vi "test_RS-xxx to GPIB ConvBox Read.vi"(8 "error in (no error)":errorcluster, 11 "TestCase in":refnum<class "Instrument Addon Serial Protocols Unit Tests.lvclass">) -> (0 "error out":errorcluster, 3 "TestCase out":refnum<class "Instrument Addon Serial Protocols Unit Tests.lvclass">)   [LabVIEW 2023, in "Instrument Addon Serial Protocols Unit Tests.lvclass"]
uses:
  Instrument Addon Serial Protocols Unit Tests.lvclass
  Instrument Addon Serial Protocols Unit Tests.lvclass/Instrument Addon Serial Protocols Unit Tests.ctl
  <vilib>/addons/_JKI Toolkits/VI Tester/TestCase.llb/TestCase.lvclass
  Listener/ListenerClassControls/Operation.ctl
  Listener/Listener.lvclass
  RS-xxx to GPIB ConvBox/RS-xxx to GPIB ConvBox.lvclass
  <vilib>/platform/TimedLoop/XDataNode/XDataNode.xnode
  <vilib>/Platform/TimedLoop/XDataNode/nitl_modes.ctl
  <vilib>/Platform/TimedLoop/XDataNode/XDNodeRunTimeDep.lvlib
  <vilib>/Platform/TimedLoop/XDataNode/wakeup.ctl
  <vilib>/Platform/TimedLoop/XDataNode/timing_clust.ctl
  Protocol Parent/Methods/Read Parameter.ctl
  Protocol Parent/Protocol Parent.lvclass
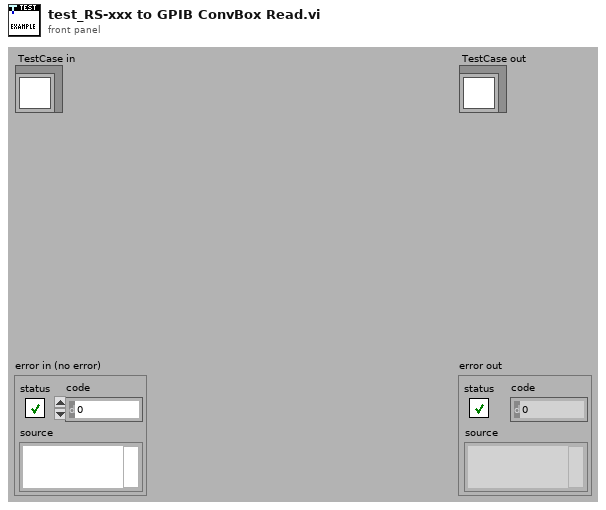
[diagram p1: front panel]
types:
  T1 = typedef "Protocols.lvlib/Protocol Parent.lvclass/Read Parameter.ctl" = cluster{"Wait Type":enum16{"Byte Count", "Wait sec"}, "Wait Value":dbl}
  T2 = typedef "Listener.lvclass/Operation.ctl" = enum16{"Read", "Write"}
  T3 = typedef "XDNodeRunTimeDep.lvlib/timing_clust.ctl" = cluster{"Expected End [f-1]":u64, "Actual End [f-1]":u64, "Finished Late? [f-1]":bool, "Expected End [i-1]":u64, "Actual End [i-1]":u64, "Finished Late? [i-1]":bool, "Expected Start [i]":u64, "Actual Start [i]":u64, "Expected Start [f]":u64, "Actual Start [f]":u64, "Source Name":string, "Structure Name":string, "Period":i64, "Deadline":i64, "Offset":i64, "Start":i64, "Priority":i32, "Timeout":i32, "Mode":T4, "Wakeup Reason":T5, "Error":errorcluster, "Source Type":string, "Secondary Source Type":string, "Global End Time":u64, "Global Start Time":u64, "Frame Duration":u64, "Iteration Duration":u64, "Assigned CPU":i32, "I/O Scan Engine Mode":u32}
  T4 = typedef "XDNodeRunTimeDep.lvlib/nitl_modes.ctl" = enum32{"No Change", "Process missed periods, maintain original phase", "Discard missed periods, maintain original phase", "Process missed periods, ignore original phase", "Discard missed periods, ignore original phase"}
  T5 = typedef "XDNodeRunTimeDep.lvlib/wakeup.ctl" = enum32{"Normal", "Aborted", "Asynchronous wakeup", "Timing source error", "Timed loop error", "Timeout"}
  T6 = typedef "Listener.lvclass/RS-xxx To GPIB ConvBox Data Structure.ctl" = cluster{"Data":string, "Command Messages Read":string[], "Address":string, "Data Length":u32}
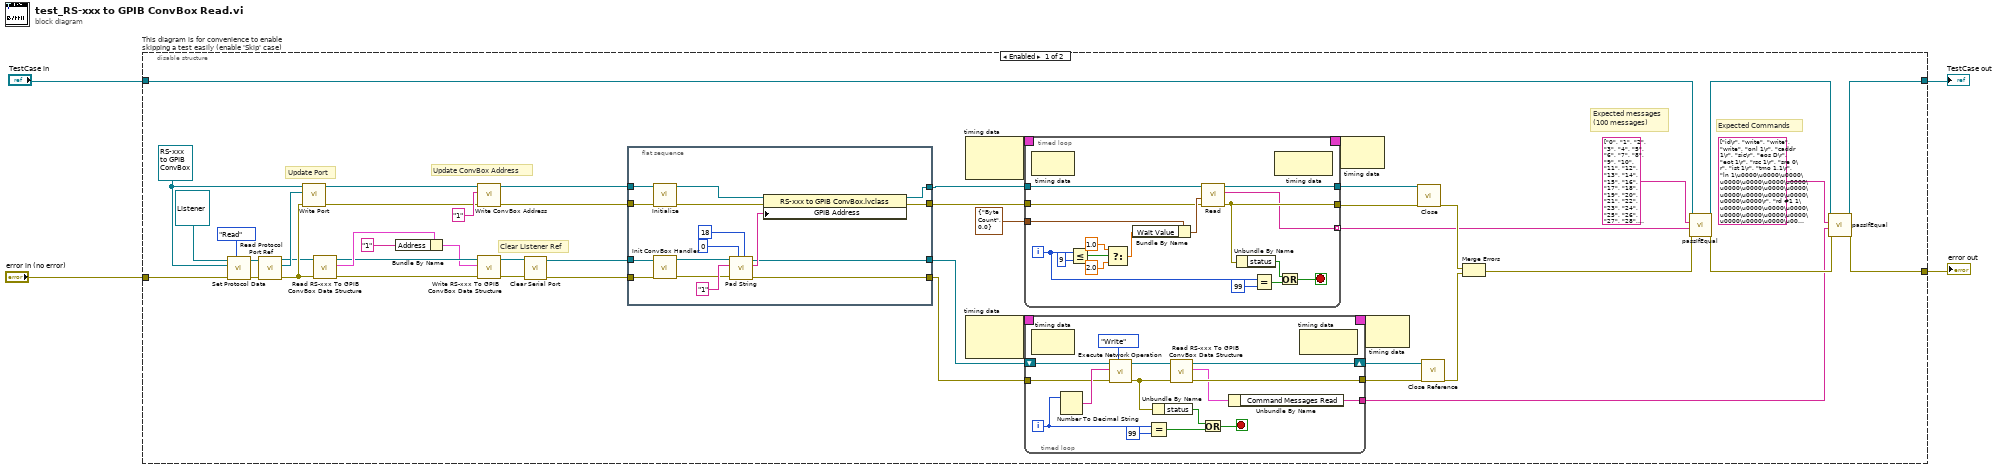
[diagram p0: block diagram]
diagram:
  n1 = disable-structure "This diagram is for convenience to enable skipping a test easily (enable 'Skip' case)" shown="Enabled" {
    disable-tunnel: "TestCase in" -> [w52 w112]
    disable-tunnel: [w10 w110] -> w1
    disable-tunnel: [w12 w111] -> w3
    disable-tunnel: "error in (no error)" -> [w51 w109]
    frame Enabled {
      w43 = refnum<class "RS-xxx to GPIB ConvBox.lvclass"> refnum ("Protocols.lvlib:RS-xxx to GPIB ConvBox.lvclass")
      # "Expected Commands"
      # "Update Port"
      # "Expected messages\n(100 messages)"
      # "Update ConvBox Address"
      # "Clear Listener Ref"
      n2 = call "Set Protocol Data.vi"("Operation"=Operation."Read", "error in (no error)"=w51, "Protocols.lvlib:Protocol Parent.lvclass"=w43, "Listener In.lvclass"=refnum<class "Listener.lvclass"> refnum ("Listener.lvclass")) -> ("error out"=w47:errorcluster, "Listener Out.lvclass"=w46:refnum<class "Listener.lvclass">)  [unwired: 6 in]
      n3 = call "Read Protocol Port Ref.vi"("error in (no error)"=w47, "Listener in"=w46) -> ("error out"=w29:errorcluster, "Protocol Port Ref"=w42:refnum<visa-resource-name>, "Listener out"=w28:refnum<class "Listener.lvclass">)  [unwired: 7 in]
      n4 = call "Write Port.vi"("error in (no error)"=w29, "Port"=w42, "RS232 to GPIB ConvBox in"=w43) -> ("error out"=w45:errorcluster, "RS232 to GPIB ConvBox out"=w44:refnum<class "RS-xxx to GPIB ConvBox.lvclass">)  [unwired: 7 in]
      n5 = call-dynamic "Read RS-xxx To GPIB ConvBox Data Structure.vi"("error in (no error)"=w29, "Listener in"=w28) -> ("error out"=w24:errorcluster, "RS-xxx To GPIB ConvBox Data Structure"=w27:T6, "Listener out"=w25:refnum<class "Listener.lvclass">)  [unwired: 7 in]
      n6 = Bundle By Name(cluster=w27, "Address"="1") -> (w23:T6)
      n7 = call "Write ConvBox Address.vi"("error in (no error)"=w45, "ConvBox Address"="1", "RS232 to GPIB ConvBox in"=w44) -> ("error out"=w8:errorcluster, "RS232 to GPIB ConvBox out"=w7:refnum<class "RS-xxx to GPIB ConvBox.lvclass">)  [unwired: 7 in]
      n8 = call-dynamic "Write RS-xxx To GPIB ConvBox Data Structure.vi"("error in (no error)"=w24, "RS-xxx To GPIB ConvBox Data Structure"=w23, "Listener in"=w25) -> ("error out"=w22:errorcluster, "Listener out"=w21:refnum<class "Listener.lvclass">)  [unwired: 7 in]
      n9 = call "Clear Serial Port.vi"("error in (no error)"=w22, "Listener In.lvclass"=w21) -> ("error out"=w6:errorcluster, "Listener out"=w5:refnum<class "Listener.lvclass">)  [unwired: 8 in]
      n10 = flat-sequence {
        tunnel: [w64] -> w20
        tunnel: [w63] -> w19
        tunnel: [w62] -> w18
        tunnel: [w61] -> w17
        tunnel: w8 -> [w60]
        tunnel: w7 -> [w59]
        tunnel: w6 -> [w56]
        tunnel: w5 -> [w55]
        frame #0 {
          n11 = call-dynamic "Initialize.vi"("error in (no error)"=w60, "RS232 to GPIB ConvBox in"=w59) -> ("error out"=w58:errorcluster, "RS232 to GPIB ConvBox out"=w57:refnum<class "RS-xxx to GPIB ConvBox.lvclass">)  [unwired: 8 in]
          n12 = call "Init ConvBox Handler.vi"("error in (no error)"=w56, "Listener in"=w55) -> ("error out"=w54:errorcluster, "Listener out"=w53:refnum<class "Listener.lvclass">)  [unwired: 8 in]
          n13 = call "Pad String.vi"("Expected Length"=u8 18, "Pad Character"=u8 0, "error in (no error)"=w54, "String To Pad"="1", "Listener in"=w53) -> ("error out"=w62:errorcluster, "Padded String"=w65:string, "Listener out"=w61:refnum<class "Listener.lvclass">)  [unwired: 4 in]
          n14 = property class="RS-xxx to GPIB ConvBox.lvclass"(reference=w57, error in=w58, "GPIB Address"=w65) -> (reference out=w63:refnum<class "RS-xxx to GPIB ConvBox.lvclass">, error out=w64:errorcluster)
        }
      }
      n15 = node-c288() -> (w41:T3)  [unwired: 2 in]
      n16 = node-c288() -> (w38:T3)  [unwired: 2 in]
      n17 = timed-loop {
        timing: w41 -> [_]
        timing-out: [_] -> w40
        tunnel: T1 {"Wait Type"=enum."Byte Count", "Wait Value"=0.0} ("Read Parameter") -> [w99]
        tunnel: [w96] -> w34
        tunnel: [w95] -> w33
        tunnel: [w94] -> w15 mode=indexing
        tunnel: w20 -> [w92]
        tunnel: w19 -> [w93]
        i -> [w90]
        stop <- w87 stop-if-true
        n18 = node-c288() -> ()  [unwired: 1 in, 1 out]
        n19 = Less Or Equal?(x=w90, y=9) -> (x <= y?=w102:bool)
        n20 = Select(t=1.0, s=w102, f=2.0) -> (s? t:f=w98:dbl)
        n21 = Bundle By Name(cluster=w99, "Wait Value"=w98) -> (w97:T1)
        n22 = call-dynamic "Read.vi"("error in (no error)"=w92, "Variant"=w97, "RS232 to GPIB ConvBox in"=w93) -> ("error out"=w96:errorcluster, "String"=w94:string, "RS232 to GPIB ConvBox out"=w95:refnum<class "RS-xxx to GPIB ConvBox.lvclass">)  [unwired: 6 in]
        n23 = Unbundle By Name(w96) -> ("status"=w91:bool)
        n24 = Equal?(x=w90, y=99) -> (x = y?=w88:bool)
        n25 = node-c288() -> ()  [unwired: 1 in, 1 out]
        n26 = Or(x=w91, y=w88) -> (x .or. y?=w87:bool)
      }
      n27 = timed-loop {
        timing: w38 -> [_]
        timing-out: [_] -> w37
        tunnel: [w71] -> w36
        tunnel: w18 -> [w81]
        tunnel: [w69] -> w13
        shift-right: [w72] -> w35
        shift-left: w17 -> [w80]
        i -> [w77]
        stop <- w78 stop-if-true
        n28 = node-c288() -> ()  [unwired: 1 in, 1 out]
        n29 = Number To Decimal String(number=w77) -> (decimal integer string=w82:string)  [unwired: 1 in]
        n30 = call "Execute Network Operation.vi"("Operation"=Operation."Write", "error in (no error)"=w81, "Message"=w82, "Listener In.lvclass"=w80) -> ("error out"=w73:errorcluster, "Listener Out.lvclass"=w74:refnum<class "Listener.lvclass">)  [unwired: 6 in]
        n31 = Equal?(x=w77, y=99) -> (x = y?=w75:bool)
        n32 = Unbundle By Name(w73) -> ("status"=w79:bool)
        n33 = call-dynamic "Read RS-xxx To GPIB ConvBox Data Structure.vi"("error in (no error)"=w73, "Listener in"=w74) -> ("error out"=w71:errorcluster, "RS-xxx To GPIB ConvBox Data Structure"=w70:T6, "Listener out"=w72:refnum<class "Listener.lvclass">)  [unwired: 7 in]
        n34 = Or(x=w79, y=w75) -> (x .or. y?=w78:bool)
        n35 = Unbundle By Name(w70) -> ("Command Messages Read"=w69:string[])
        n36 = node-c288() -> ()  [unwired: 1 in, 1 out]
      }
      n37 = node-c288(w40) -> ()  [unwired: 1 out]
      n38 = node-c288(w37) -> ()  [unwired: 1 out]
      n39 = call-dynamic "Close.vi"("error in (no error)"=w34, "RS232 to GPIB ConvBox in"=w33) -> ("error out"=w32:errorcluster)  [unwired: 8 in, 1 out]
      n40 = call "Close Reference.vi"("error in (no error)"=w36, "Listener In.lvclass"=w35) -> ("error out"=w31:errorcluster)  [unwired: 8 in, 1 out]
      n41 = Merge Errors(w32, w31) -> (w30:errorcluster)
      n42 = call-dynamic "passIfEqual.vi"("error in (no error)"=w30, "y"=w15, "x"=string[] ["0", "1", "2", "3", "4", "5", "6", "7", "8", "9", "10", "11", "12", "13", "14", "15", "16", "17", "18", "19", "20", "21", "22", "23", "24", "25", "26", "27", "28", "29", "30", "31", "32", "33", "34", "35", "36", "37", "38", "39", "40", "41", "42", "43", "44", "45", "46", "47", "48", "49", "50", "51", "52", "53", "54", "55", "56", "57", "58", "59", "60", "61", "62", "63", "64", "65", "66", "67", "68", "69", "70", "71", "72", "73", "74", "75", "76", "77", "78", "79", "80", "81", "82", "83", "84", "85", "86", "87", "88", "89", "90", "91", "92", "93", "94", "95", "96", "97", "98", "99"] ("Array"), "TestCase in"=w52) -> ("error out"=w14:errorcluster, "TestCase out"=w11:refnum<class "Instrument Addon Serial Protocols Unit Tests.lvclass">)  [unwired: 6 in]
      n43 = call-dynamic "passIfEqual.vi"("error in (no error)"=w14, "y"=w13, "x"=string[] ["id\r", "write", "write", "write", "onl 1\r", "caddr 1\r", "sic\r", "eos D\r", "eot 1\r", "rsc 1\r", "sre 0\r", "ist 1\r", "tmo 1,1\r", "ln 1\u0000\u0000\u0000\u0000\u0000\u0000\u0000\u0000\u0000\u0000\u0000\u0000\u0000\u0000\u0000\u0000\u0000\r", "rd #1 1\u0000\u0000\u0000\u0000\u0000\u0000\u0000\u0000\u0000\u0000\u0000\u0000\u0000\u0000\u0000\u0000\u0000\r", "stat n\r", "ln 1\u0000\u0000\u0000\u0000\u0000\u0000\u0000\u0000\u0000\u0000\u0000\u0000\u0000\u0000\u0000\u0000\u0000\r", "rd #1 1\u0000\u0000\u0000\u0000\u0000\u0000\u0000\u0000\u0000\u0000\u0000\u0000\u0000\u0000\u0000\u0000\u0000\r", "stat n\r", "ln 1\u0000\u0000\u0000\u0000\u0000\u0000\u0000\u0000\u0000\u0000\u0000\u0000\u0000\u0000\u0000\u0000\u0000\r", "rd #1 1\u0000\u0000\u0000\u0000\u0000\u0000\u0000\u0000\u0000\u0000\u0000\u0000\u0000\u0000\u0000\u0000\u0000\r", "stat n\r", "ln 1\u0000\u0000\u0000\u0000\u0000\u0000\u0000\u0000\u0000\u0000\u0000\u0000\u0000\u0000\u0000\u0000\u0000\r", "rd #1 1\u0000\u0000\u0000\u0000\u0000\u0000\u0000\u0000\u0000\u0000\u0000\u0000\u0000\u0000\u0000\u0000\u0000\r", "stat n\r", "ln 1\u0000\u0000\u0000\u0000\u0000\u0000\u0000\u0000\u0000\u0000\u0000\u0000\u0000\u0000\u0000\u0000\u0000\r", "rd #1 1\u0000\u0000\u0000\u0000\u0000\u0000\u0000\u0000\u0000\u0000\u0000\u0000\u0000\u0000\u0000\u0000\u0000\r", "stat n\r", "ln 1\u0000\u0000\u0000\u0000\u0000\u0000\u0000\u0000\u0000\u0000\u0000\u0000\u0000\u0000\u0000\u0000\u0000\r", "rd #1 1\u0000\u0000\u0000\u0000\u0000\u0000\u0000\u0000\u0000\u0000\u0000\u0000\u0000\u0000\u0000\u0000\u0000\r", "stat n\r", "ln 1\u0000\u0000\u0000\u0000\u0000\u0000\u0000\u0000\u0000\u0000\u0000\u0000\u0000\u0000\u0000\u0000\u0000\r", "rd #1 1\u0000\u0000\u0000\u0000\u0000\u0000\u0000\u0000\u0000\u0000\u0000\u0000\u0000\u0000\u0000\u0000\u0000\r", "stat n\r", "ln 1\u0000\u0000\u0000\u0000\u0000\u0000\u0000\u0000\u0000\u0000\u0000\u0000\u0000\u0000\u0000\u0000\u0000\r", "rd #1 1\u0000\u0000\u0000\u0000\u0000\u0000\u0000\u0000\u0000\u0000\u0000\u0000\u0000\u0000\u0000\u0000\u0000\r", "stat n\r", "ln 1\u0000\u0000\u0000\u0000\u0000\u0000\u0000\u0000\u0000\u0000\u0000\u0000\u0000\u0000\u0000\u0000\u0000\r", "rd #1 1\u0000\u0000\u0000\u0000\u0000\u0000\u0000\u0000\u0000\u0000\u0000\u0000\u0000\u0000\u0000\u0000\u0000\r", "stat n\r", "ln 1\u0000\u0000\u0000\u0000\u0000\u0000\u0000\u0000\u0000\u0000\u0000\u0000\u0000\u0000\u0000\u0000\u0000\r", "rd #1 1\u0000\u0000\u0000\u0000\u0000\u0000\u0000\u0000\u0000\u0000\u0000\u0000\u0000\u0000\u0000\u0000\u0000\r", "stat n\r", "ln 1\u0000\u0000\u0000\u0000\u0000\u0000\u0000\u0000\u0000\u0000\u0000\u0000\u0000\u0000\u0000\u0000\u0000\r", "rd #2 1\u0000\u0000\u0000\u0000\u0000\u0000\u0000\u0000\u0000\u0000\u0000\u0000\u0000\u0000\u0000\u0000\u0000\r", "stat n\r", "ln 1\u0000\u0000\u0000\u0000\u0000\u0000\u0000\u0000\u0000\u0000\u0000\u0000\u0000\u0000\u0000\u0000\u0000\r", "rd #2 1\u0000\u0000\u0000\u0000\u0000\u0000\u0000\u0000\u0000\u0000\u0000\u0000\u0000\u0000\u0000\u0000\u0000\r", "stat n\r", "ln 1\u0000\u0000\u0000\u0000\u0000\u0000\u0000\u0000\u0000\u0000\u0000\u0000\u0000\u0000\u0000\u0000\u0000\r", "rd #2 1\u0000\u0000\u0000\u0000\u0000\u0000\u0000\u0000\u0000\u0000\u0000\u0000\u0000\u0000\u0000\u0000\u0000\r", "stat n\r", "ln 1\u0000\u0000\u0000\u0000\u0000\u0000\u0000\u0000\u0000\u0000\u0000\u0000\u0000\u0000\u0000\u0000\u0000\r", "rd #2 1\u0000\u0000\u0000\u0000\u0000\u0000\u0000\u0000\u0000\u0000\u0000\u0000\u0000\u0000\u0000\u0000\u0000\r", "stat n\r", "ln 1\u0000\u0000\u0000\u0000\u0000\u0000\u0000\u0000\u0000\u0000\u0000\u0000\u0000\u0000\u0000\u0000\u0000\r", "rd #2 1\u0000\u0000\u0000\u0000\u0000\u0000\u0000\u0000\u0000\u0000\u0000\u0000\u0000\u0000\u0000\u0000\u0000\r", "stat n\r", "ln 1\u0000\u0000\u0000\u0000\u0000\u0000\u0000\u0000\u0000\u0000\u0000\u0000\u0000\u0000\u0000\u0000\u0000\r", "rd #2 1\u0000\u0000\u0000\u0000\u0000\u0000\u0000\u0000\u0000\u0000\u0000\u0000\u0000\u0000\u0000\u0000\u0000\r", "stat n\r", "ln 1\u0000\u0000\u0000\u0000\u0000\u0000\u0000\u0000\u0000\u0000\u0000\u0000\u0000\u0000\u0000\u0000\u0000\r", "rd #2 1\u0000\u0000\u0000\u0000\u0000\u0000\u0000\u0000\u0000\u0000\u0000\u0000\u0000\u0000\u0000\u0000\u0000\r", "stat n\r", "ln 1\u0000\u0000\u0000\u0000\u0000\u0000\u0000\u0000\u0000\u0000\u0000\u0000\u0000\u0000\u0000\u0000\u0000\r", "rd #2 1\u0000\u0000\u0000\u0000\u0000\u0000\u0000\u0000\u0000\u0000\u0000\u0000\u0000\u0000\u0000\u0000\u0000\r", "stat n\r", "ln 1\u0000\u0000\u0000\u0000\u0000\u0000\u0000\u0000\u0000\u0000\u0000\u0000\u0000\u0000\u0000\u0000\u0000\r", "rd #2 1\u0000\u0000\u0000\u0000\u0000\u0000\u0000\u0000\u0000\u0000\u0000\u0000\u0000\u0000\u0000\u0000\u0000\r", "stat n\r", "ln 1\u0000\u0000\u0000\u0000\u0000\u0000\u0000\u0000\u0000\u0000\u0000\u0000\u0000\u0000\u0000\u0000\u0000\r", "rd #2 1\u0000\u0000\u0000\u0000\u0000\u0000\u0000\u0000\u0000\u0000\u0000\u0000\u0000\u0000\u0000\u0000\u0000\r", "stat n\r", "ln 1\u0000\u0000\u0000\u0000\u0000\u0000\u0000\u0000\u0000\u0000\u0000\u0000\u0000\u0000\u0000\u0000\u0000\r", "rd #2 1\u0000\u0000\u0000\u0000\u0000\u0000\u0000\u0000\u0000\u0000\u0000\u0000\u0000\u0000\u0000\u0000\u0000\r", "stat n\r", "ln 1\u0000\u0000\u0000\u0000\u0000\u0000\u0000\u0000\u0000\u0000\u0000\u0000\u0000\u0000\u0000\u0000\u0000\r", "rd #2 1\u0000\u0000\u0000\u0000\u0000\u0000\u0000\u0000\u0000\u0000\u0000\u0000\u0000\u0000\u0000\u0000\u0000\r", "stat n\r", "ln 1\u0000\u0000\u0000\u0000\u0000\u0000\u0000\u0000\u0000\u0000\u0000\u0000\u0000\u0000\u0000\u0000\u0000\r", "rd #2 1\u0000\u0000\u0000\u0000\u0000\u0000\u0000\u0000\u0000\u0000\u0000\u0000\u0000\u0000\u0000\u0000\u0000\r", "stat n\r", "ln 1\u0000\u0000\u0000\u0000\u0000\u0000\u0000\u0000\u0000\u0000\u0000\u0000\u0000\u0000\u0000\u0000\u0000\r", "rd #2 1\u0000\u0000\u0000\u0000\u0000\u0000\u0000\u0000\u0000\u0000\u0000\u0000\u0000\u0000\u0000\u0000\u0000\r", "stat n\r", "ln 1\u0000\u0000\u0000\u0000\u0000\u0000\u0000\u0000\u0000\u0000\u0000\u0000\u0000\u0000\u0000\u0000\u0000\r", "rd #2 1\u0000\u0000\u0000\u0000\u0000\u0000\u0000\u0000\u0000\u0000\u0000\u0000\u0000\u0000\u0000\u0000\u0000\r", "stat n\r", "ln 1\u0000\u0000\u0000\u0000\u0000\u0000\u0000\u0000\u0000\u0000\u0000\u0000\u0000\u0000\u0000\u0000\u0000\r", "rd #2 1\u0000\u0000\u0000\u0000\u0000\u0000\u0000\u0000\u0000\u0000\u0000\u0000\u0000\u0000\u0000\u0000\u0000\r", "stat n\r", "ln 1\u0000\u0000\u0000\u0000\u0000\u0000\u0000\u0000\u0000\u0000\u0000\u0000\u0000\u0000\u0000\u0000\u0000\r", "rd #2 1\u0000\u0000\u0000\u0000\u0000\u0000\u0000\u0000\u0000\u0000\u0000\u0000\u0000\u0000\u0000\u0000\u0000\r", "stat n\r", "ln 1\u0000\u0000\u0000\u0000\u0000\u0000\u0000\u0000\u0000\u0000\u0000\u0000\u0000\u0000\u0000\u0000\u0000\r", "rd #2 1\u0000\u0000\u0000\u0000\u0000\u0000\u0000\u0000\u0000\u0000\u0000\u0000\u0000\u0000\u0000\u0000\u0000\r", "stat n\r", "ln 1\u0000\u0000\u0000\u0000\u0000\u0000\u0000\u0000\u0000\u0000\u0000\u0000\u0000\u0000\u0000\u0000\u0000\r", "rd #2 1\u0000\u0000\u0000\u0000\u0000\u0000\u0000\u0000\u0000\u0000\u0000\u0000\u0000\u0000\u0000\u0000\u0000\r", "stat n\r", "ln 1\u0000\u0000\u0000\u0000\u0000\u0000\u0000\u0000\u0000\u0000\u0000\u0000\u0000\u0000\u0000\u0000\u0000\r", "rd #2 1\u0000\u0000\u0000\u0000\u0000\u0000\u0000\u0000\u0000\u0000\u0000\u0000\u0000\u0000\u0000\u0000\u0000\r", "stat n\r", "ln 1\u0000\u0000\u0000\u0000\u0000\u0000\u0000\u0000\u0000\u0000\u0000\u0000\u0000\u0000\u0000\u0000\u0000\r", "rd #2 1\u0000\u0000\u0000\u0000\u0000\u0000\u0000\u0000\u0000\u0000\u0000\u0000\u0000\u0000\u0000\u0000\u0000\r", "stat n\r", "ln 1\u0000\u0000\u0000\u0000\u0000\u0000\u0000\u0000\u0000\u0000\u0000\u0000\u0000\u0000\u0000\u0000\u0000\r", "rd #2 1\u0000\u0000\u0000\u0000\u0000\u0000\u0000\u0000\u0000\u0000\u0000\u0000\u0000\u0000\u0000\u0000\u0000\r", "stat n\r", "ln 1\u0000\u0000\u0000\u0000\u0000\u0000\u0000\u0000\u0000\u0000\u0000\u0000\u0000\u0000\u0000\u0000\u0000\r", "rd #2 1\u0000\u0000\u0000\u0000\u0000\u0000\u0000\u0000\u0000\u0000\u0000\u0000\u0000\u0000\u0000\u0000\u0000\r", "stat n\r", "ln 1\u0000\u0000\u0000\u0000\u0000\u0000\u0000\u0000\u0000\u0000\u0000\u0000\u0000\u0000\u0000\u0000\u0000\r", "rd #2 1\u0000\u0000\u0000\u0000\u0000\u0000\u0000\u0000\u0000\u0000\u0000\u0000\u0000\u0000\u0000\u0000\u0000\r", "stat n\r", "ln 1\u0000\u0000\u0000\u0000\u0000\u0000\u0000\u0000\u0000\u0000\u0000\u0000\u0000\u0000\u0000\u0000\u0000\r", "rd #2 1\u0000\u0000\u0000\u0000\u0000\u0000\u0000\u0000\u0000\u0000\u0000\u0000\u0000\u0000\u0000\u0000\u0000\r", "stat n\r", "ln 1\u0000\u0000\u0000\u0000\u0000\u0000\u0000\u0000\u0000\u0000\u0000\u0000\u0000\u0000\u0000\u0000\u0000\r", "rd #2 1\u0000\u0000\u0000\u0000\u0000\u0000\u0000\u0000\u0000\u0000\u0000\u0000\u0000\u0000\u0000\u0000\u0000\r", "stat n\r", "ln 1\u0000\u0000\u0000\u0000\u0000\u0000\u0000\u0000\u0000\u0000\u0000\u0000\u0000\u0000\u0000\u0000\u0000\r", "rd #2 1\u0000\u0000\u0000\u0000\u0000\u0000\u0000\u0000\u0000\u0000\u0000\u0000\u0000\u0000\u0000\u0000\u0000\r", "stat n\r", "ln 1\u0000\u0000\u0000\u0000\u0000\u0000\u0000\u0000\u0000\u0000\u0000\u0000\u0000\u0000\u0000\u0000\u0000\r", "rd #2 1\u0000\u0000\u0000\u0000\u0000\u0000\u0000\u0000\u0000\u0000\u0000\u0000\u0000\u0000\u0000\u0000\u0000\r", "stat n\r", "ln 1\u0000\u0000\u0000\u0000\u0000\u0000\u0000\u0000\u0000\u0000\u0000\u0000\u0000\u0000\u0000\u0000\u0000\r", "rd #2 1\u0000\u0000\u0000\u0000\u0000\u0000\u0000\u0000\u0000\u0000\u0000\u0000\u0000\u0000\u0000\u0000\u0000\r", "stat n\r", "ln 1\u0000\u0000\u0000\u0000\u0000\u0000\u0000\u0000\u0000\u0000\u0000\u0000\u0000\u0000\u0000\u0000\u0000\r", "rd #2 1\u0000\u0000\u0000\u0000\u0000\u0000\u0000\u0000\u0000\u0000\u0000\u0000\u0000\u0000\u0000\u0000\u0000\r", "stat n\r", "ln 1\u0000\u0000\u0000\u0000\u0000\u0000\u0000\u0000\u0000\u0000\u0000\u0000\u0000\u0000\u0000\u0000\u0000\r", "rd #2 1\u0000\u0000\u0000\u0000\u0000\u0000\u0000\u0000\u0000\u0000\u0000\u0000\u0000\u0000\u0000\u0000\u0000\r", "stat n\r", "ln 1\u0000\u0000\u0000\u0000\u0000\u0000\u0000\u0000\u0000\u0000\u0000\u0000\u0000\u0000\u0000\u0000\u0000\r", "rd #2 1\u0000\u0000\u0000\u0000\u0000\u0000\u0000\u0000\u0000\u0000\u0000\u0000\u0000\u0000\u0000\u0000\u0000\r", "stat n\r", "ln 1\u0000\u0000\u0000\u0000\u0000\u0000\u0000\u0000\u0000\u0000\u0000\u0000\u0000\u0000\u0000\u0000\u0000\r", "rd #2 1\u0000\u0000\u0000\u0000\u0000\u0000\u0000\u0000\u0000\u0000\u0000\u0000\u0000\u0000\u0000\u0000\u0000\r", "stat n\r", "ln 1\u0000\u0000\u0000\u0000\u0000\u0000\u0000\u0000\u0000\u0000\u0000\u0000\u0000\u0000\u0000\u0000\u0000\r", "rd #2 1\u0000\u0000\u0000\u0000\u0000\u0000\u0000\u0000\u0000\u0000\u0000\u0000\u0000\u0000\u0000\u0000\u0000\r", "stat n\r", "ln 1\u0000\u0000\u0000\u0000\u0000\u0000\u0000\u0000\u0000\u0000\u0000\u0000\u0000\u0000\u0000\u0000\u0000\r", "rd #2 1\u0000\u0000\u0000\u0000\u0000\u0000\u0000\u0000\u0000\u0000\u0000\u0000\u0000\u0000\u0000\u0000\u0000\r", "stat n\r", "ln 1\u0000\u0000\u0000\u0000\u0000\u0000\u0000\u0000\u0000\u0000\u0000\u0000\u0000\u0000\u0000\u0000\u0000\r", "rd #2 1\u0000\u0000\u0000\u0000\u0000\u0000\u0000\u0000\u0000\u0000\u0000\u0000\u0000\u0000\u0000\u0000\u0000\r", "stat n\r", "ln 1\u0000\u0000\u0000\u0000\u0000\u0000\u0000\u0000\u0000\u0000\u0000\u0000\u0000\u0000\u0000\u0000\u0000\r", "rd #2 1\u0000\u0000\u0000\u0000\u0000\u0000\u0000\u0000\u0000\u0000\u0000\u0000\u0000\u0000\u0000\u0000\u0000\r", "stat n\r", "ln 1\u0000\u0000\u0000\u0000\u0000\u0000\u0000\u0000\u0000\u0000\u0000\u0000\u0000\u0000\u0000\u0000\u0000\r", "rd #2 1\u0000\u0000\u0000\u0000\u0000\u0000\u0000\u0000\u0000\u0000\u0000\u0000\u0000\u0000\u0000\u0000\u0000\r", "stat n\r", "ln 1\u0000\u0000\u0000\u0000\u0000\u0000\u0000\u0000\u0000\u0000\u0000\u0000\u0000\u0000\u0000\u0000\u0000\r", "rd #2 1\u0000\u0000\u0000\u0000\u0000\u0000\u0000\u0000\u0000\u0000\u0000\u0000\u0000\u0000\u0000\u0000\u0000\r", "stat n\r", "ln 1\u0000\u0000\u0000\u0000\u0000\u0000\u0000\u0000\u0000\u0000\u0000\u0000\u0000\u0000\u0000\u0000\u0000\r", "rd #2 1\u0000\u0000\u0000\u0000\u0000\u0000\u0000\u0000\u0000\u0000\u0000\u0000\u0000\u0000\u0000\u0000\u0000\r", "stat n\r", "ln 1\u0000\u0000\u0000\u0000\u0000\u0000\u0000\u0000\u0000\u0000\u0000\u0000\u0000\u0000\u0000\u0000\u0000\r", "rd #2 1\u0000\u0000\u0000\u0000\u0000\u0000\u0000\u0000\u0000\u0000\u0000\u0000\u0000\u0000\u0000\u0000\u0000\r", "stat n\r", "ln 1\u0000\u0000\u0000\u0000\u0000\u0000\u0000\u0000\u0000\u0000\u0000\u0000\u0000\u0000\u0000\u0000\u0000\r", "rd #2 1\u0000\u0000\u0000\u0000\u0000\u0000\u0000\u0000\u0000\u0000\u0000\u0000\u0000\u0000\u0000\u0000\u0000\r", "stat n\r", "ln 1\u0000\u0000\u0000\u0000\u0000\u0000\u0000\u0000\u0000\u0000\u0000\u0000\u0000\u0000\u0000\u0000\u0000\r", "rd #2 1\u0000\u0000\u0000\u0000\u0000\u0000\u0000\u0000\u0000\u0000\u0000\u0000\u0000\u0000\u0000\u0000\u0000\r", "stat n\r", "ln 1\u0000\u0000\u0000\u0000\u0000\u0000\u0000\u0000\u0000\u0000\u0000\u0000\u0000\u0000\u0000\u0000\u0000\r", "rd #2 1\u0000\u0000\u0000\u0000\u0000\u0000\u0000\u0000\u0000\u0000\u0000\u0000\u0000\u0000\u0000\u0000\u0000\r", "stat n\r", "ln 1\u0000\u0000\u0000\u0000\u0000\u0000\u0000\u0000\u0000\u0000\u0000\u0000\u0000\u0000\u0000\u0000\u0000\r", "rd #2 1\u0000\u0000\u0000\u0000\u0000\u0000\u0000\u0000\u0000\u0000\u0000\u0000\u0000\u0000\u0000\u0000\u0000\r", "stat n\r", "ln 1\u0000\u0000\u0000\u0000\u0000\u0000\u0000\u0000\u0000\u0000\u0000\u0000\u0000\u0000\u0000\u0000\u0000\r", "rd #2 1\u0000\u0000\u0000\u0000\u0000\u0000\u0000\u0000\u0000\u0000\u0000\u0000\u0000\u0000\u0000\u0000\u0000\r", "stat n\r", "ln 1\u0000\u0000\u0000\u0000\u0000\u0000\u0000\u0000\u0000\u0000\u0000\u0000\u0000\u0000\u0000\u0000\u0000\r", "rd #2 1\u0000\u0000\u0000\u0000\u0000\u0000\u0000\u0000\u0000\u0000\u0000\u0000\u0000\u0000\u0000\u0000\u0000\r", "stat n\r", "ln 1\u0000\u0000\u0000\u0000\u0000\u0000\u0000\u0000\u0000\u0000\u0000\u0000\u0000\u0000\u0000\u0000\u0000\r", "rd #2 1\u0000\u0000\u0000\u0000\u0000\u0000\u0000\u0000\u0000\u0000\u0000\u0000\u0000\u0000\u0000\u0000\u0000\r", "stat n\r", "ln 1\u0000\u0000\u0000\u0000\u0000\u0000\u0000\u0000\u0000\u0000\u0000\u0000\u0000\u0000\u0000\u0000\u0000\r", "rd #2 1\u0000\u0000\u0000\u0000\u0000\u0000\u0000\u0000\u0000\u0000\u0000\u0000\u0000\u0000\u0000\u0000\u0000\r", "stat n\r", "ln 1\u0000\u0000\u0000\u0000\u0000\u0000\u0000\u0000\u0000\u0000\u0000\u0000\u0000\u0000\u0000\u0000\u0000\r", "rd #2 1\u0000\u0000\u0000\u0000\u0000\u0000\u0000\u0000\u0000\u0000\u0000\u0000\u0000\u0000\u0000\u0000\u0000\r", "stat n\r", "ln 1\u0000\u0000\u0000\u0000\u0000\u0000\u0000\u0000\u0000\u0000\u0000\u0000\u0000\u0000\u0000\u0000\u0000\r", "rd #2 1\u0000\u0000\u0000\u0000\u0000\u0000\u0000\u0000\u0000\u0000\u0000\u0000\u0000\u0000\u0000\u0000\u0000\r", "stat n\r", "ln 1\u0000\u0000\u0000\u0000\u0000\u0000\u0000\u0000\u0000\u0000\u0000\u0000\u0000\u0000\u0000\u0000\u0000\r", "rd #2 1\u0000\u0000\u0000\u0000\u0000\u0000\u0000\u0000\u0000\u0000\u0000\u0000\u0000\u0000\u0000\u0000\u0000\r", "stat n\r", "ln 1\u0000\u0000\u0000\u0000\u0000\u0000\u0000\u0000\u0000\u0000\u0000\u0000\u0000\u0000\u0000\u0000\u0000\r", "rd #2 1\u0000\u0000\u0000\u0000\u0000\u0000\u0000\u0000\u0000\u0000\u0000\u0000\u0000\u0000\u0000\u0000\u0000\r", "stat n\r", "ln 1\u0000\u0000\u0000\u0000\u0000\u0000\u0000\u0000\u0000\u0000\u0000\u0000\u0000\u0000\u0000\u0000\u0000\r", "rd #2 1\u0000\u0000\u0000\u0000\u0000\u0000\u0000\u0000\u0000\u0000\u0000\u0000\u0000\u0000\u0000\u0000\u0000\r", "stat n\r", "ln 1\u0000\u0000\u0000\u0000\u0000\u0000\u0000\u0000\u0000\u0000\u0000\u0000\u0000\u0000\u0000\u0000\u0000\r", "rd #2 1\u0000\u0000\u0000\u0000\u0000\u0000\u0000\u0000\u0000\u0000\u0000\u0000\u0000\u0000\u0000\u0000\u0000\r", "stat n\r", "ln 1\u0000\u0000\u0000\u0000\u0000\u0000\u0000\u0000\u0000\u0000\u0000\u0000\u0000\u0000\u0000\u0000\u0000\r", "rd #2 1\u0000\u0000\u0000\u0000\u0000\u0000\u0000\u0000\u0000\u0000\u0000\u0000\u0000\u0000\u0000\u0000\u0000\r", "stat n\r", "ln 1\u0000\u0000\u0000\u0000\u0000\u0000\u0000\u0000\u0000\u0000\u0000\u0000\u0000\u0000\u0000\u0000\u0000\r", "rd #2 1\u0000\u0000\u0000\u0000\u0000\u0000\u0000\u0000\u0000\u0000\u0000\u0000\u0000\u0000\u0000\u0000\u0000\r", "stat n\r", "ln 1\u0000\u0000\u0000\u0000\u0000\u0000\u0000\u0000\u0000\u0000\u0000\u0000\u0000\u0000\u0000\u0000\u0000\r", "rd #2 1\u0000\u0000\u0000\u0000\u0000\u0000\u0000\u0000\u0000\u0000\u0000\u0000\u0000\u0000\u0000\u0000\u0000\r", "stat n\r", "ln 1\u0000\u0000\u0000\u0000\u0000\u0000\u0000\u0000\u0000\u0000\u0000\u0000\u0000\u0000\u0000\u0000\u0000\r", "rd #2 1\u0000\u0000\u0000\u0000\u0000\u0000\u0000\u0000\u0000\u0000\u0000\u0000\u0000\u0000\u0000\u0000\u0000\r", "stat n\r", "ln 1\u0000\u0000\u0000\u0000\u0000\u0000\u0000\u0000\u0000\u0000\u0000\u0000\u0000\u0000\u0000\u0000\u0000\r", "rd #2 1\u0000\u0000\u0000\u0000\u0000\u0000\u0000\u0000\u0000\u0000\u0000\u0000\u0000\u0000\u0000\u0000\u0000\r", "stat n\r", "ln 1\u0000\u0000\u0000\u0000\u0000\u0000\u0000\u0000\u0000\u0000\u0000\u0000\u0000\u0000\u0000\u0000\u0000\r", "rd #2 1\u0000\u0000\u0000\u0000\u0000\u0000\u0000\u0000\u0000\u0000\u0000\u0000\u0000\u0000\u0000\u0000\u0000\r", "stat n\r", "ln 1\u0000\u0000\u0000\u0000\u0000\u0000\u0000\u0000\u0000\u0000\u0000\u0000\u0000\u0000\u0000\u0000\u0000\r", "rd #2 1\u0000\u0000\u0000\u0000\u0000\u0000\u0000\u0000\u0000\u0000\u0000\u0000\u0000\u0000\u0000\u0000\u0000\r", "stat n\r", "ln 1\u0000\u0000\u0000\u0000\u0000\u0000\u0000\u0000\u0000\u0000\u0000\u0000\u0000\u0000\u0000\u0000\u0000\r", "rd #2 1\u0000\u0000\u0000\u0000\u0000\u0000\u0000\u0000\u0000\u0000\u0000\u0000\u0000\u0000\u0000\u0000\u0000\r", "stat n\r", "ln 1\u0000\u0000\u0000\u0000\u0000\u0000\u0000\u0000\u0000\u0000\u0000\u0000\u0000\u0000\u0000\u0000\u0000\r", "rd #2 1\u0000\u0000\u0000\u0000\u0000\u0000\u0000\u0000\u0000\u0000\u0000\u0000\u0000\u0000\u0000\u0000\u0000\r", "stat n\r", "ln 1\u0000\u0000\u0000\u0000\u0000\u0000\u0000\u0000\u0000\u0000\u0000\u0000\u0000\u0000\u0000\u0000\u0000\r", "rd #2 1\u0000\u0000\u0000\u0000\u0000\u0000\u0000\u0000\u0000\u0000\u0000\u0000\u0000\u0000\u0000\u0000\u0000\r", "stat n\r", "ln 1\u0000\u0000\u0000\u0000\u0000\u0000\u0000\u0000\u0000\u0000\u0000\u0000\u0000\u0000\u0000\u0000\u0000\r", "rd #2 1\u0000\u0000\u0000\u0000\u0000\u0000\u0000\u0000\u0000\u0000\u0000\u0000\u0000\u0000\u0000\u0000\u0000\r", "stat n\r", "ln 1\u0000\u0000\u0000\u0000\u0000\u0000\u0000\u0000\u0000\u0000\u0000\u0000\u0000\u0000\u0000\u0000\u0000\r", "rd #2 1\u0000\u0000\u0000\u0000\u0000\u0000\u0000\u0000\u0000\u0000\u0000\u0000\u0000\u0000\u0000\u0000\u0000\r", "stat n\r", "ln 1\u0000\u0000\u0000\u0000\u0000\u0000\u0000\u0000\u0000\u0000\u0000\u0000\u0000\u0000\u0000\u0000\u0000\r", "rd #2 1\u0000\u0000\u0000\u0000\u0000\u0000\u0000\u0000\u0000\u0000\u0000\u0000\u0000\u0000\u0000\u0000\u0000\r", "stat n\r", "ln 1\u0000\u0000\u0000\u0000\u0000\u0000\u0000\u0000\u0000\u0000\u0000\u0000\u0000\u0000\u0000\u0000\u0000\r", "rd #2 1\u0000\u0000\u0000\u0000\u0000\u0000\u0000\u0000\u0000\u0000\u0000\u0000\u0000\u0000\u0000\u0000\u0000\r", "stat n\r", "ln 1\u0000\u0000\u0000\u0000\u0000\u0000\u0000\u0000\u0000\u0000\u0000\u0000\u0000\u0000\u0000\u0000\u0000\r", "rd #2 1\u0000\u0000\u0000\u0000\u0000\u0000\u0000\u0000\u0000\u0000\u0000\u0000\u0000\u0000\u0000\u0000\u0000\r", "stat n\r", "ln 1\u0000\u0000\u0000\u0000\u0000\u0000\u0000\u0000\u0000\u0000\u0000\u0000\u0000\u0000\u0000\u0000\u0000\r", "rd #2 1\u0000\u0000\u0000\u0000\u0000\u0000\u0000\u0000\u0000\u0000\u0000\u0000\u0000\u0000\u0000\u0000\u0000\r", "stat n\r", "ln 1\u0000\u0000\u0000\u0000\u0000\u0000\u0000\u0000\u0000\u0000\u0000\u0000\u0000\u0000\u0000\u0000\u0000\r", "rd #2 1\u0000\u0000\u0000\u0000\u0000\u0000\u0000\u0000\u0000\u0000\u0000\u0000\u0000\u0000\u0000\u0000\u0000\r", "stat n\r", "ln 1\u0000\u0000\u0000\u0000\u0000\u0000\u0000\u0000\u0000\u0000\u0000\u0000\u0000\u0000\u0000\u0000\u0000\r", "rd #2 1\u0000\u0000\u0000\u0000\u0000\u0000\u0000\u0000\u0000\u0000\u0000\u0000\u0000\u0000\u0000\u0000\u0000\r", "stat n\r", "ln 1\u0000\u0000\u0000\u0000\u0000\u0000\u0000\u0000\u0000\u0000\u0000\u0000\u0000\u0000\u0000\u0000\u0000\r", "rd #2 1\u0000\u0000\u0000\u0000\u0000\u0000\u0000\u0000\u0000\u0000\u0000\u0000\u0000\u0000\u0000\u0000\u0000\r", "stat n\r", "ln 1\u0000\u0000\u0000\u0000\u0000\u0000\u0000\u0000\u0000\u0000\u0000\u0000\u0000\u0000\u0000\u0000\u0000\r", "rd #2 1\u0000\u0000\u0000\u0000\u0000\u0000\u0000\u0000\u0000\u0000\u0000\u0000\u0000\u0000\u0000\u0000\u0000\r", "stat n\r", "ln 1\u0000\u0000\u0000\u0000\u0000\u0000\u0000\u0000\u0000\u0000\u0000\u0000\u0000\u0000\u0000\u0000\u0000\r", "rd #2 1\u0000\u0000\u0000\u0000\u0000\u0000\u0000\u0000\u0000\u0000\u0000\u0000\u0000\u0000\u0000\u0000\u0000\r", "stat n\r", "ln 1\u0000\u0000\u0000\u0000\u0000\u0000\u0000\u0000\u0000\u0000\u0000\u0000\u0000\u0000\u0000\u0000\u0000\r", "rd #2 1\u0000\u0000\u0000\u0000\u0000\u0000\u0000\u0000\u0000\u0000\u0000\u0000\u0000\u0000\u0000\u0000\u0000\r", "stat n\r", "ln 1\u0000\u0000\u0000\u0000\u0000\u0000\u0000\u0000\u0000\u0000\u0000\u0000\u0000\u0000\u0000\u0000\u0000\r", "rd #2 1\u0000\u0000\u0000\u0000\u0000\u0000\u0000\u0000\u0000\u0000\u0000\u0000\u0000\u0000\u0000\u0000\u0000\r", "stat n\r", "ln 1\u0000\u0000\u0000\u0000\u0000\u0000\u0000\u0000\u0000\u0000\u0000\u0000\u0000\u0000\u0000\u0000\u0000\r", "rd #2 1\u0000\u0000\u0000\u0000\u0000\u0000\u0000\u0000\u0000\u0000\u0000\u0000\u0000\u0000\u0000\u0000\u0000\r", "stat n\r", "ln 1\u0000\u0000\u0000\u0000\u0000\u0000\u0000\u0000\u0000\u0000\u0000\u0000\u0000\u0000\u0000\u0000\u0000\r", "rd #2 1\u0000\u0000\u0000\u0000\u0000\u0000\u0000\u0000\u0000\u0000\u0000\u0000\u0000\u0000\u0000\u0000\u0000\r", "stat n\r", "ln 1\u0000\u0000\u0000\u0000\u0000\u0000\u0000\u0000\u0000\u0000\u0000\u0000\u0000\u0000\u0000\u0000\u0000\r", "rd #2 1\u0000\u0000\u0000\u0000\u0000\u0000\u0000\u0000\u0000\u0000\u0000\u0000\u0000\u0000\u0000\u0000\u0000\r", "stat n\r", "ln 1\u0000\u0000\u0000\u0000\u0000\u0000\u0000\u0000\u0000\u0000\u0000\u0000\u0000\u0000\u0000\u0000\u0000\r", "rd #2 1\u0000\u0000\u0000\u0000\u0000\u0000\u0000\u0000\u0000\u0000\u0000\u0000\u0000\u0000\u0000\u0000\u0000\r", "stat n\r", "ln 1\u0000\u0000\u0000\u0000\u0000\u0000\u0000\u0000\u0000\u0000\u0000\u0000\u0000\u0000\u0000\u0000\u0000\r", "rd #2 1\u0000\u0000\u0000\u0000\u0000\u0000\u0000\u0000\u0000\u0000\u0000\u0000\u0000\u0000\u0000\u0000\u0000\r", "stat n\r", "ln 1\u0000\u0000\u0000\u0000\u0000\u0000\u0000\u0000\u0000\u0000\u0000\u0000\u0000\u0000\u0000\u0000\u0000\r", "rd #2 1\u0000\u0000\u0000\u0000\u0000\u0000\u0000\u0000\u0000\u0000\u0000\u0000\u0000\u0000\u0000\u0000\u0000\r", "stat n\r", "ln 1\u0000\u0000\u0000\u0000\u0000\u0000\u0000\u0000\u0000\u0000\u0000\u0000\u0000\u0000\u0000\u0000\u0000\r", "rd #2 1\u0000\u0000\u0000\u0000\u0000\u0000\u0000\u0000\u0000\u0000\u0000\u0000\u0000\u0000\u0000\u0000\u0000\r", "stat n\r", "ln 1\u0000\u0000\u0000\u0000\u0000\u0000\u0000\u0000\u0000\u0000\u0000\u0000\u0000\u0000\u0000\u0000\u0000\r", "rd #2 1\u0000\u0000\u0000\u0000\u0000\u0000\u0000\u0000\u0000\u0000\u0000\u0000\u0000\u0000\u0000\u0000\u0000\r", "stat n\r", "ln 1\u0000\u0000\u0000\u0000\u0000\u0000\u0000\u0000\u0000\u0000\u0000\u0000\u0000\u0000\u0000\u0000\u0000\r", "rd #2 1\u0000\u0000\u0000\u0000\u0000\u0000\u0000\u0000\u0000\u0000\u0000\u0000\u0000\u0000\u0000\u0000\u0000\r", "stat n\r", "ln 1\u0000\u0000\u0000\u0000\u0000\u0000\u0000\u0000\u0000\u0000\u0000\u0000\u0000\u0000\u0000\u0000\u0000\r", "rd #2 1\u0000\u0000\u0000\u0000\u0000\u0000\u0000\u0000\u0000\u0000\u0000\u0000\u0000\u0000\u0000\u0000\u0000\r", "stat n\r", "ln 1\u0000\u0000\u0000\u0000\u0000\u0000\u0000\u0000\u0000\u0000\u0000\u0000\u0000\u0000\u0000\u0000\u0000\r", "rd #2 1\u0000\u0000\u0000\u0000\u0000\u0000\u0000\u0000\u0000\u0000\u0000\u0000\u0000\u0000\u0000\u0000\u0000\r", "stat n\r", "ln 1\u0000\u0000\u0000\u0000\u0000\u0000\u0000\u0000\u0000\u0000\u0000\u0000\u0000\u0000\u0000\u0000\u0000\r", "rd #2 1\u0000\u0000\u0000\u0000\u0000\u0000\u0000\u0000\u0000\u0000\u0000\u0000\u0000\u0000\u0000\u0000\u0000\r", "stat n\r"] ("Command Messages Read"), "TestCase in"=w11) -> ("error out"=w12:errorcluster, "TestCase out"=w10:refnum<class "Instrument Addon Serial Protocols Unit Tests.lvclass">)  [unwired: 6 in]
    }
    frame Disabled {
      # "skip test result while test is under development"
      n44 = call <vilib>:"skip.vi"("error in (no error)"=w109, "TestCase in"=w112) -> ("error out"=w111:errorcluster, "TestCase out"=w110:refnum<class "Instrument Addon Serial Protocols Unit Tests.lvclass">)  [unwired: 8 in]
    }
  }
  "error out" <- w3
  "TestCase out" <- w1
